vi "Status download.vi"(8 "error in (no error)":errorcluster, 10 "replies":string[](array[string]), 11 "Motor in":refnum<class "Motor.lvclass">) -> (0 "error out":errorcluster, 1 "error":bool, 2 "status":T1, 3 "Motor out":refnum<class "Motor.lvclass">)   [LabVIEW 2018, in "Motor.lvclass"]
uses:
  Motor.lvclass
  Motor.lvclass/Motor.ctl
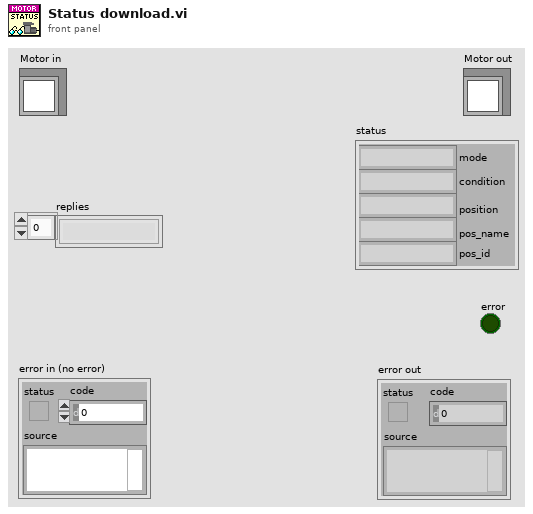
[diagram p1: front panel]
types:
  T1 = cluster{"mode":string, "condition":string, "position":string, "pos_name":string, "pos_id":string}
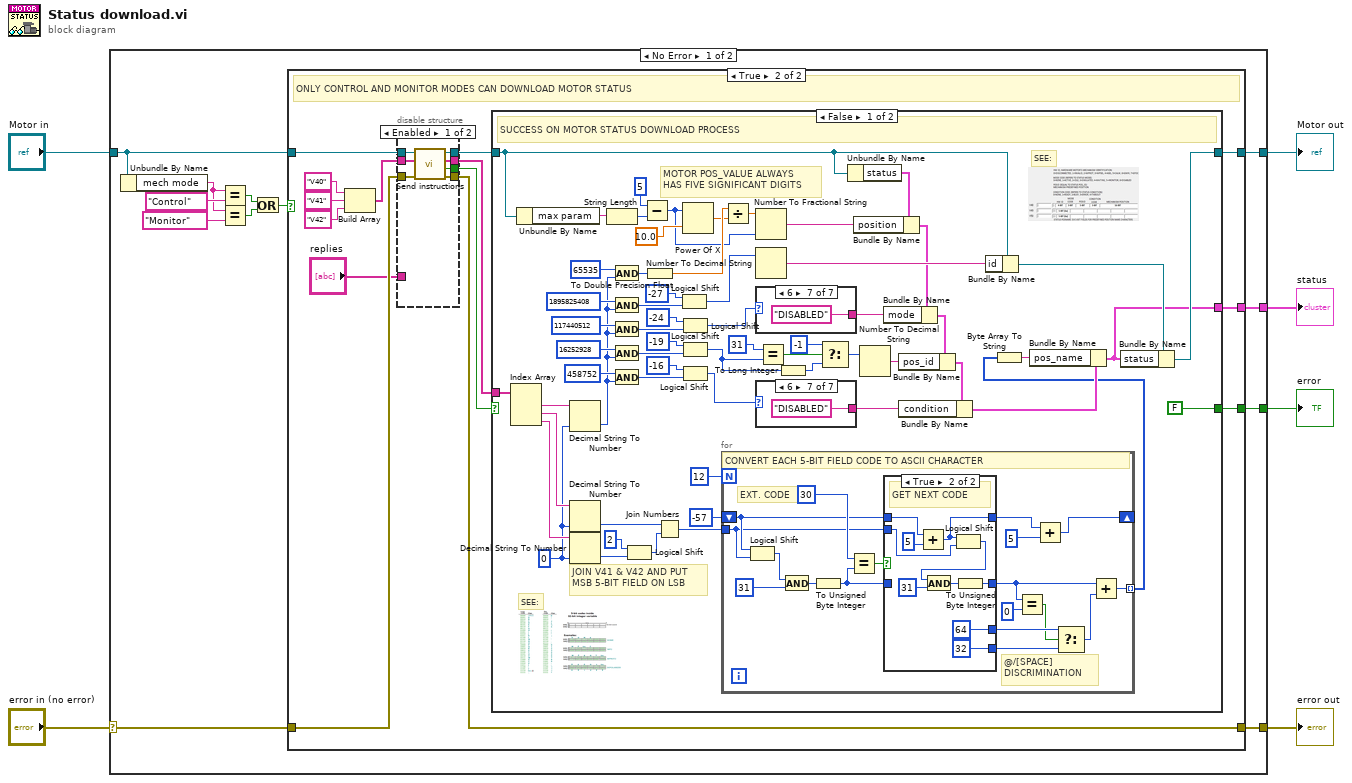
[diagram p0: block diagram]
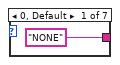
[diagram p4: hidden frame]
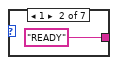
[diagram p5: hidden frame]
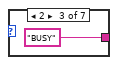
[diagram p6: hidden frame]
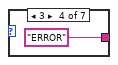
[diagram p7: hidden frame]
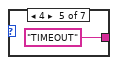
[diagram p8: hidden frame]
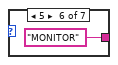
[diagram p9: hidden frame]
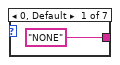
[diagram p10: hidden frame]
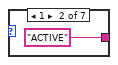
[diagram p11: hidden frame]
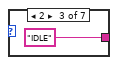
[diagram p12: hidden frame]
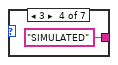
[diagram p13: hidden frame]
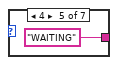
[diagram p14: hidden frame]
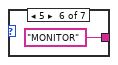
[diagram p15: hidden frame]
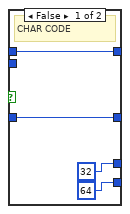
[diagram p16: hidden frame]
diagram:
  n1 = case shown="No Error" "error in (no error)" {
    selector: "error in (no error)" -> [w11 w154]
    tunnel: [w10 w154] -> w5
    tunnel: [w7 w155] -> w3
    tunnel: "Motor in" -> [w12 w155]
    tunnel: [w9 _] -> w2
    tunnel: [w8 _] -> w1
    frame No Error {
      n2 = Unbundle By Name(w12) -> ("mech mode"=w16:string)
      n3 = Equal?(x=w16, y="Control" ("GF mode")) -> (x = y?=w14:bool)
      n4 = Equal?(x=w16, y="Monitor" ("GF mode")) -> (x = y?=w15:bool)
      n5 = Or(x=w14, y=w15) -> (x .or. y?=w13:bool)
      n6 = case shown="True" w13 {
        tunnel: w12 -> [w20 w31]
        tunnel: [w20 w25] -> w7
        tunnel: w11 -> [w19 w29]
        tunnel: [w19 w24] -> w10
        tunnel: [_ w23] -> w9
        tunnel: [_ w22] -> w8
        frame False {
          # "NONE AND SIMULATED MODES DO NOT DOWNLOAD MOTOR STATUS"
        }
        frame True {
          # "ONLY CONTROL AND MONITOR MODES CAN DOWNLOAD MOTOR STATUS"
          n7 = Build Array("V40", "V41", "V42") -> (w30:string[])
          n8 = disable-structure shown="Enabled" {
            disable-tunnel: w31 -> [w41 w42]
            disable-tunnel: w30 -> [w40 _]
            disable-tunnel: w29 -> [w39 w44]
            disable-tunnel: [w38 w43] -> w28
            disable-tunnel: [w37 _] -> w27
            disable-tunnel: [w36 w42] -> w26
            disable-tunnel: [w35 w44] -> w24
            disable-tunnel: "replies" -> [_ w43]
            frame Enabled {
              n9 = call-dynamic "Send instructions.vi"("error in (no error)"=w39, "instructions"=w40, "Motor in"=w41) -> ("error out"=w35:errorcluster, "error"=w37:bool, "replies"=w38:string[], "Motor out"=w36:refnum<class "Motor.lvclass">)  [unwired: 4 in, 1 out]
            }
            frame Disabled {
            }
          }
          n10 = case shown="False" w27 {
            selector: w27 -> [_ w152]
            tunnel: w28 -> [w105 _]
            tunnel: w26 -> [w63 w153]
            tunnel: [w61 w153] -> w25
            tunnel: [FALSE w152] -> w23
            tunnel: [w59 _] -> w22
            frame False {
              w96 = u32 0 ("default (0 I32)")
              # "MOTOR POS_VALUE ALWAYS\nHAS FIVE SIGNIFICANT DIGITS"
              # "SEE:"
              # "SEE:"
              # "JOIN V41 & V42 AND PUT\nMSB 5-BIT FIELD ON LSB"
              # "SUCCESS ON MOTOR STATUS DOWNLOAD PROCESS"
              n11 = Index Array(array=w105) -> (element #1=w97:string, element #2=w104:string, element #3=w103:string)  [unwired: 3 in]
              n12 = Unbundle By Name(w63) -> ("max param"=w80:string)
              n13 = Decimal String To Number(string=w97, default (0L)=w96) -> (number=w58:u32)  [unwired: 1 in, 1 out]
              n14 = Decimal String To Number(string=w104, default (0L)=w96) -> (number=w102:u32)  [unwired: 1 in, 1 out]
              n15 = Decimal String To Number(string=w103, default (0L)=w96) -> (number=w101:u32)  [unwired: 1 in, 1 out]
              n16 = String Length(string=w80) -> (length=w81:i32)
              n17 = And(x=u32 65535, y=w58) -> (x .and. y?=w83:u32)
              n18 = And(x=u32 1895825408, y=w58) -> (x .and. y?=w89:u32)
              n19 = And(x=u32 117440512, y=w58) -> (x .and. y?=w87:u32)
              n20 = And(x=u32 16252928, y=w58) -> (x .and. y?=w85:u32)
              n21 = And(x=u32 458752, y=w58) -> (x .and. y?=w74:u32)
              n22 = Logical Shift(y=i16 2, x=w101) -> (x << y=w99:u32)
              n23 = Subtract(x=5 ("x-y"), y=w81) -> (x-y=w75:i32)
              n24 = To Double Precision Float(number=w83) -> (double precision float=w79:dbl)
              n25 = Join Numbers(hi=w102, lo=w99) -> ((hi.lo)=w54:u64)
              n26 = Logical Shift(y=i16 -27, x=w89) -> (x << y=w55:u32)
              n27 = Logical Shift(y=i16 -24, x=w87) -> (x << y=w56:u32)
              n28 = Logical Shift(y=i16 -19, x=w85) -> (x << y=w45:u32)
              n29 = Logical Shift(y=i16 -16, x=w74) -> (x << y=w57:u32)
              n30 = Power Of X(1:10.0 ("x"), 2:w75) -> (0:w78:dbl)
              n31 = for {
                N: 12 -> [_]
                tunnel: [w135] -> w51 mode=indexing
                tunnel: w54 -> [w130]
                shift-right: [w127] -> _
                shift-left: i16 -57 ("y") -> [w132]
                # "@/[SPACE]\nDISCRIMINATION"
                # "EXT. CODE"
                # "CONVERT EACH 5-BIT FIELD CODE TO ASCII CHARACTER"
                n32 = Logical Shift(y=w132, x=w130) -> (x << y=w131:u64)
                n33 = And(x=w131, y=u64 31) -> (x .and. y?=w136:u64)
                n34 = To Unsigned Byte Integer(number=w136) -> (unsigned 8bit integer=w129:u8)
                n35 = Equal?(x=u8 30 ("unsigned 8bit integer"), y=w129) -> (x = y?=w133:bool)
                n36 = case shown="True" w133 {
                  tunnel: w132 -> [w140 w145]
                  tunnel: w130 -> [_ w151]
                  tunnel: w129 -> [w141 _]
                  tunnel: [w141 w148] -> w124
                  tunnel: [w140 w142] -> w126
                  tunnel: [u8 32 ("unsigned 8bit integer") u8 64 ("unsigned 8bit integer")] -> w123
                  tunnel: [u8 64 ("unsigned 8bit integer") u8 32 ("unsigned 8bit integer")] -> w122
                  frame False {
                    # "CHAR CODE"
                  }
                  frame True {
                    # "GET NEXT CODE"
                    n37 = Add(x=w145, y=i16 5) -> (x+y=w142:i16)
                    n38 = Logical Shift(y=w142, x=w151) -> (x << y=w146:u64)
                    n39 = And(x=w146, y=u64 31) -> (x .and. y?=w150:u64)
                    n40 = To Unsigned Byte Integer(number=w150) -> (unsigned 8bit integer=w148:u8)
                  }
                }
                n41 = Equal?(x=w124, y=u8 0) -> (x = y?=w121:bool)
                n42 = Add(x=w126, y=i16 5) -> (x+y=w127:i16)
                n43 = Select(t=w123, s=w121, f=w122) -> (s? t:f=w120:u8)
                n44 = Add(x=w124, y=w120) -> (x+y=w135:u8)
              }
              n45 = Divide(x=w79, y=w78) -> (x/y=w76:dbl)
              n46 = Number To Fractional String(number=w76, precision (6)=w75) -> (F-format string=w71:string)  [unwired: 2 in]
              n47 = Number To Decimal String(number=w55) -> (decimal integer string=w70:string)  [unwired: 1 in]
              n48 = case shown="6" w56 {
                tunnel: ["NONE" "ACTIVE" "IDLE" "SIMULATED" "WAITING" "MONITOR" "DISABLED"] -> w73
                frame 0, Default {
                }
                frame 1 {
                }
                frame 2 {
                }
                frame 3 {
                }
                frame 4 {
                }
                frame 5 {
                }
                frame 6 {
                }
              }
              n49 = case shown="6" w57 {
                tunnel: ["NONE" "READY" "BUSY" "ERROR" "TIMEOUT" "MONITOR" "DISABLED"] -> w72
                frame 0, Default {
                }
                frame 1 {
                }
                frame 2 {
                }
                frame 3 {
                }
                frame 4 {
                }
                frame 5 {
                }
                frame 6 {
                }
              }
              n50 = Equal?(x=u32 31 ("default (0 I32)"), y=w45) -> (x = y?=w50:bool)
              n51 = To Long Integer(number=w45) -> (32bit integer=w46:i32)
              n52 = Select(t=-1 ("default (0 I32)"), s=w50, f=w46) -> (s? t:f=w49:i32)
              n53 = Unbundle By Name(w63) -> ("status"=w68:T1)
              n54 = Bundle By Name(cluster=w68, "position"=w71) -> (w67:T1)
              n55 = Number To Decimal String(number=w49) -> (decimal integer string=w69:string)  [unwired: 1 in]
              n56 = Bundle By Name(cluster=w67, "mode"=w73) -> (w66:T1)
              n57 = Bundle By Name(cluster=w66, "pos_id"=w69) -> (w65:T1)
              n58 = Bundle By Name(cluster=w65, "condition"=w72) -> (w64:T1)
              n59 = Bundle By Name(cluster=w63, "id"=w70) -> (w62:refnum<class "Motor.lvclass">)
              n60 = Byte Array To String(unsigned byte array=w51) -> (string=w52:string)
              n61 = Bundle By Name(cluster=w64, "pos_name"=w52) -> (w59:T1)
              n62 = Bundle By Name(cluster=w62, "status"=w59) -> (w61:refnum<class "Motor.lvclass">)
            }
            frame True {
              # "ERROR ON MOTOR STATUS DOWNLOAD PROCESS"
            }
          }
        }
      }
    }
    frame Error {
    }
  }
  "error out" <- w5
  "Motor out" <- w3
  "status" <- w1
  "error" <- w2
